vi "动态优化复测判定2.vi"(10 "T1-T2":dbl[](array[numeric]) format="%#.6f", 11 "Vres":dbl[](array[numeric]) format="%#.6f") -> (3 "结果1":bool)   [LabVIEW 2020]
uses:
  Global_Variable/Global.vi
  Global_Variable/A180648.vi
  <userlib>/_MGI/1D Array/MGI Average/MGI Average (DBL[]).vi
panel:
  out "结果2":bool
  out "结果3":bool
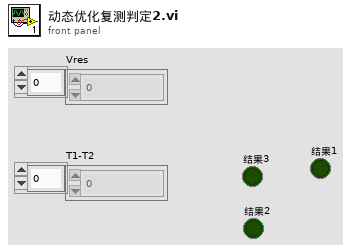
[diagram p1: front panel]
types:
  T1 = cluster{"主副信号合格范围":cluster{"单位":string, "下限":dbl, "上限":dbl}, "可信度合格范围":cluster{"单位":string, "下限":dbl, "上限":dbl}, "主副信号差差值":cluster{"单位":string, "下限":dbl, "上限":dbl}, "静态T1-T2范围":cluster{"单位":string, "下限":dbl, "上限":dbl}, "静态T1-T2偏差范围":cluster{"单位":string, "下限":dbl, "上限":dbl}}
  T2 = cluster{"曲线范围":cluster{"单位":string, "角度下限":dbl, "角度上限":dbl}}
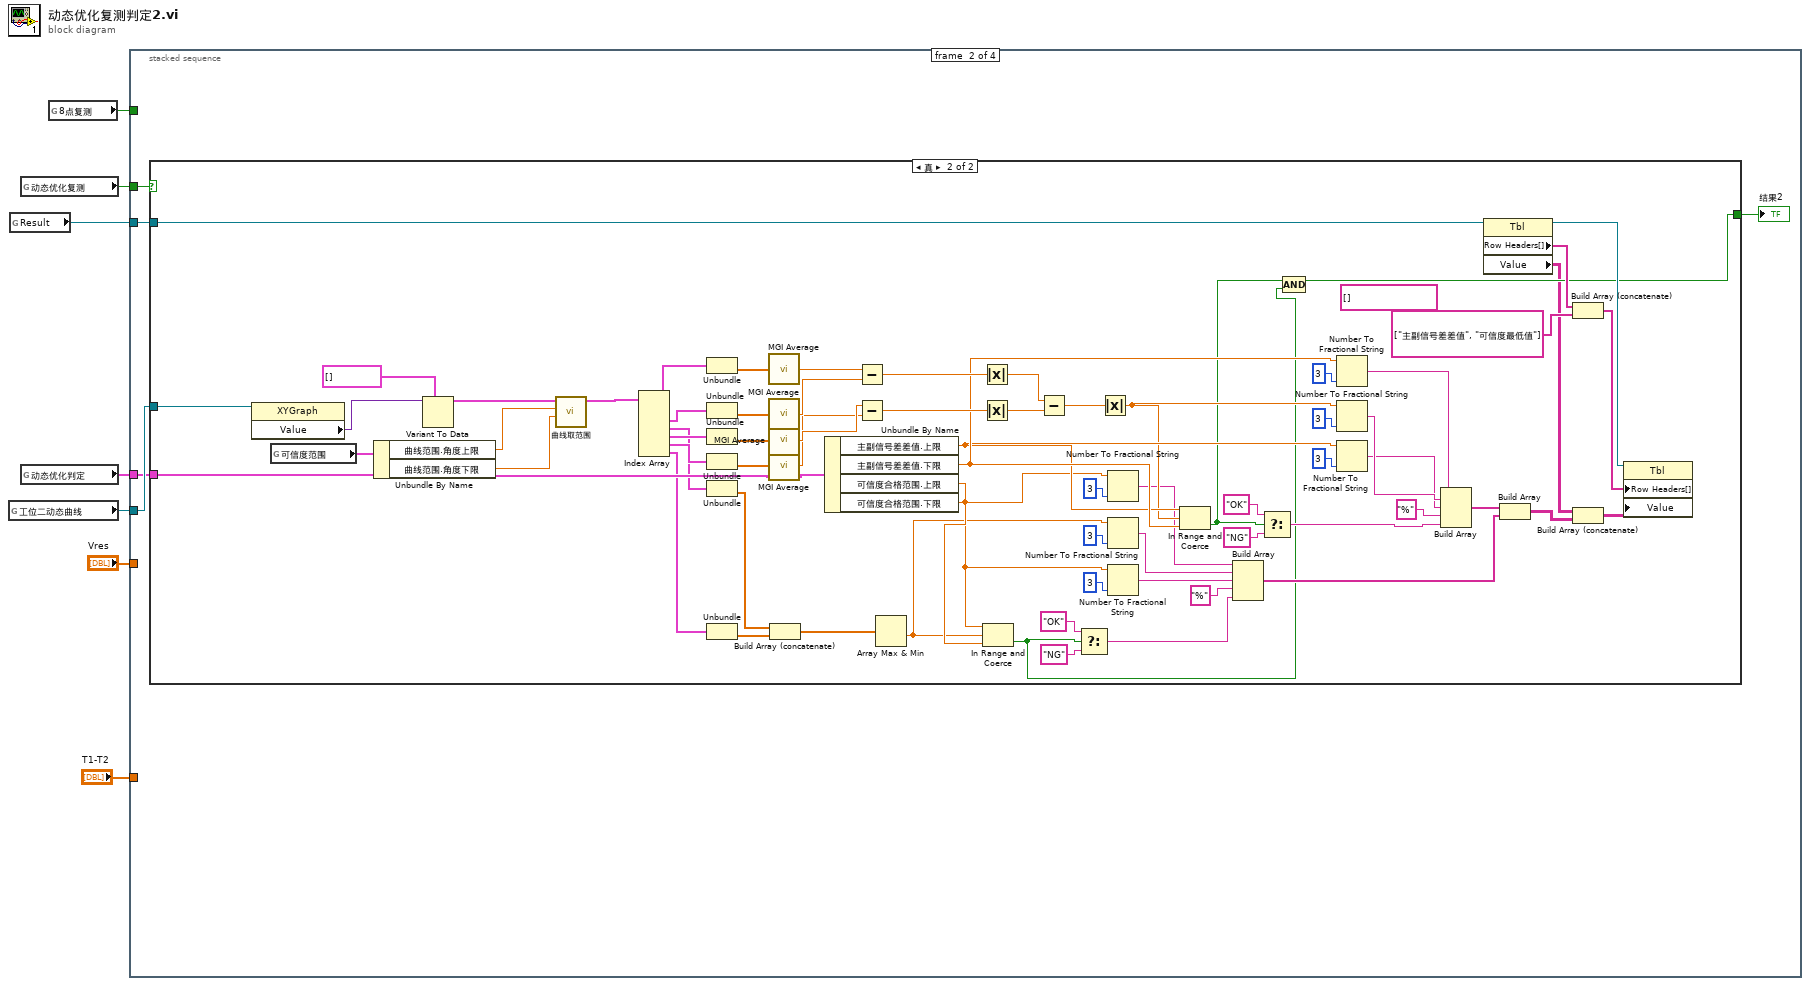
[diagram p0: block diagram]
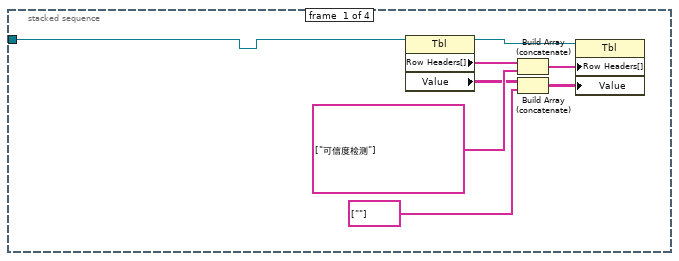
[diagram p2: hidden frame]
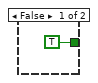
[diagram p3: hidden frame]
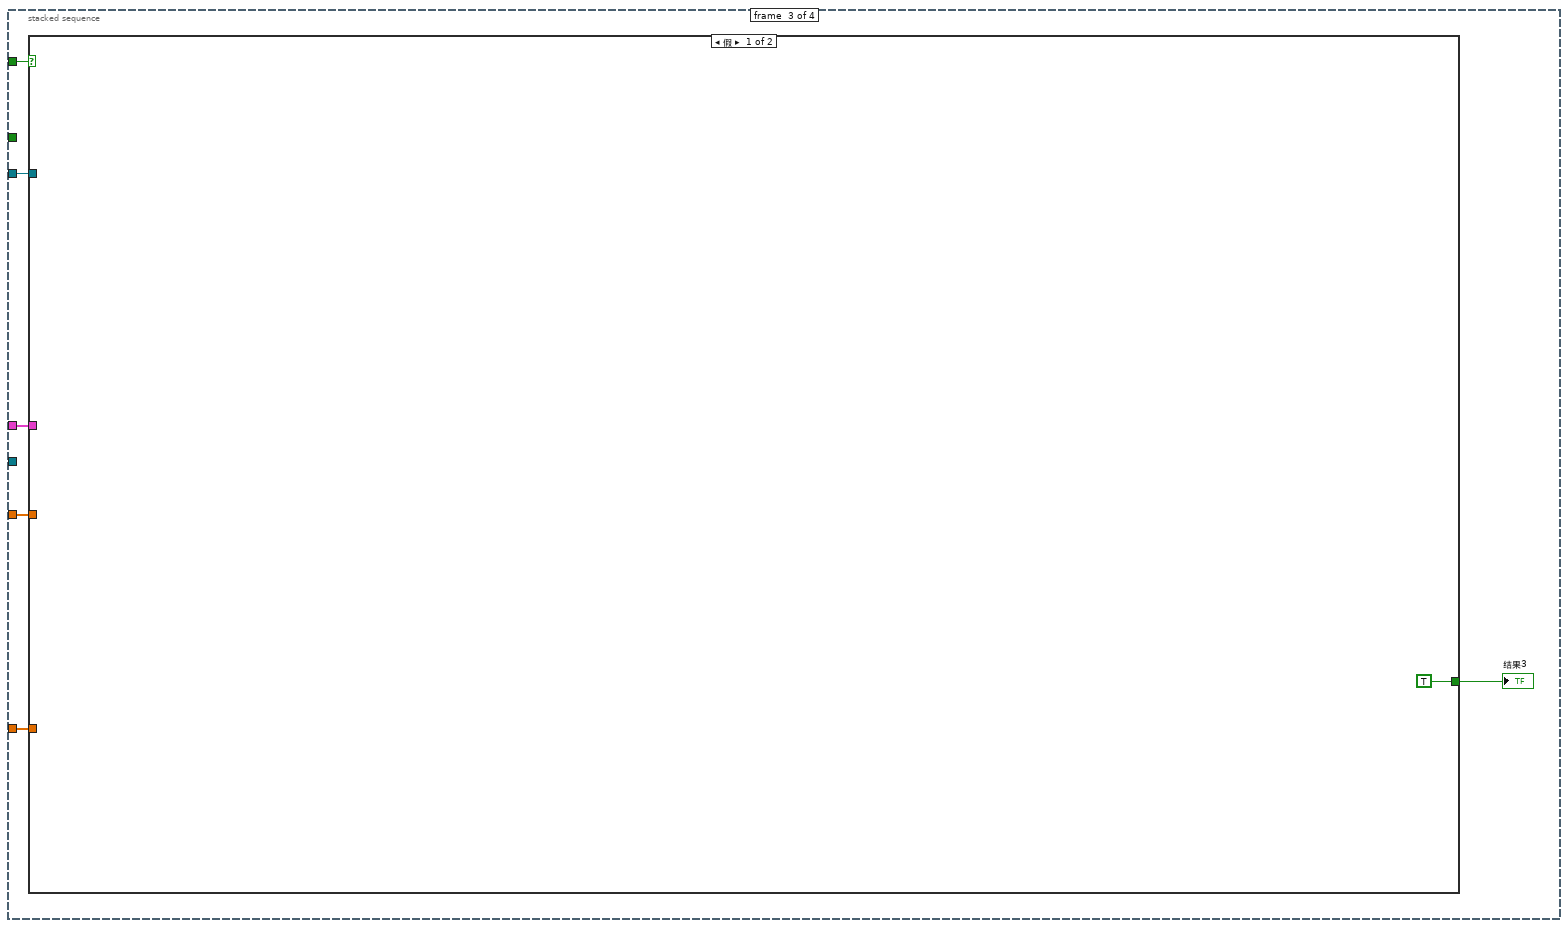
[diagram p4: hidden frame]
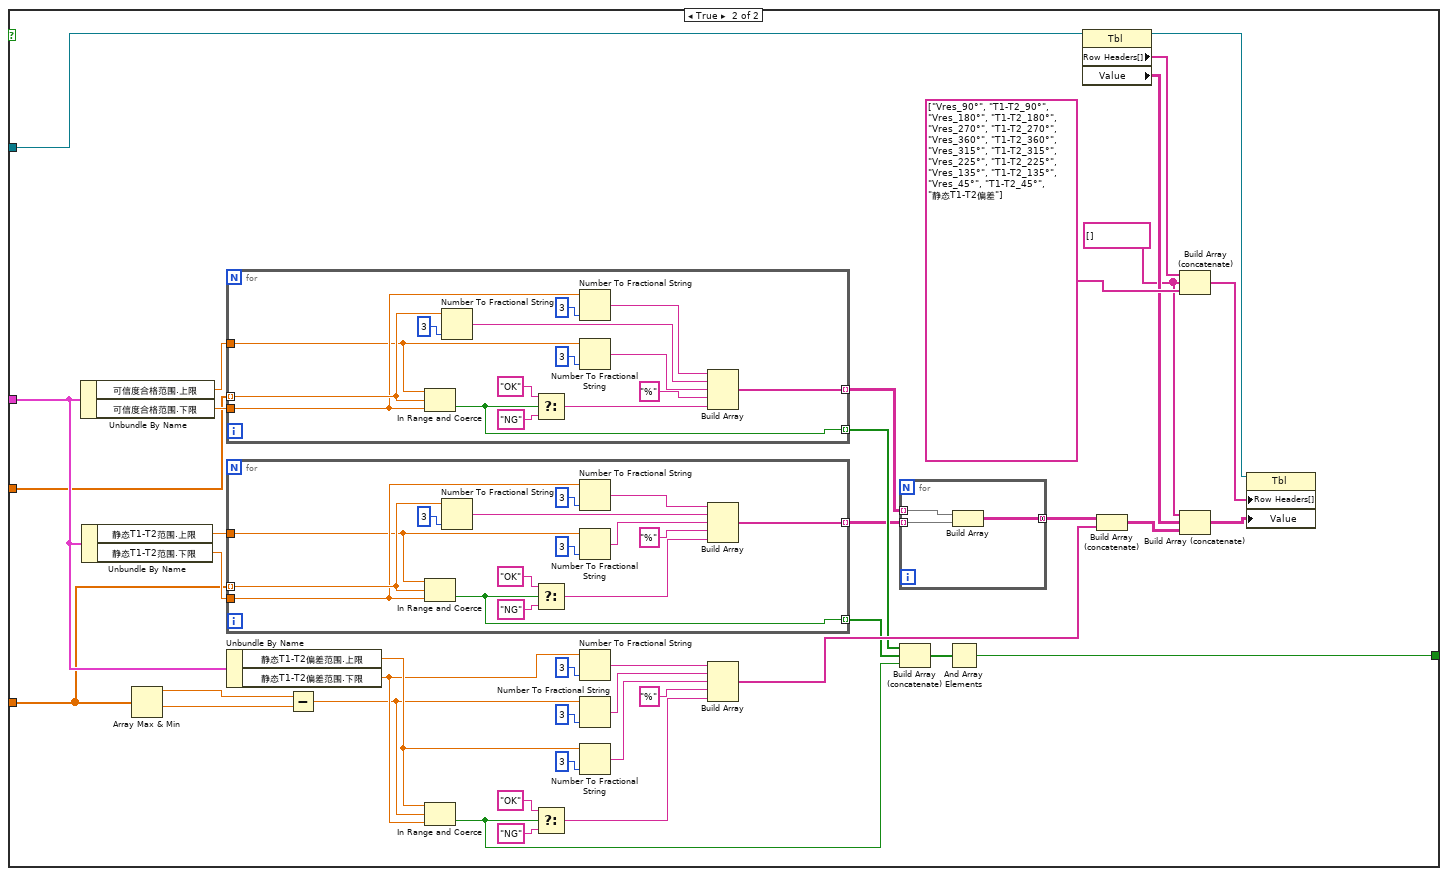
[diagram p5: hidden frame]
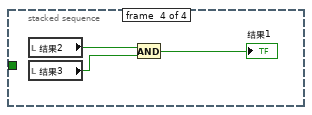
[diagram p6: hidden frame]
diagram:
  n1 = global read "A180648.vi" "工位二动态曲线"() -> (w6:refnum<vi>)
  n2 = global read "Global.vi" "Result"() -> (w1:refnum<vi>)
  n3 = global read "Global.vi" "动态优化复测"() -> (w3:bool)
  n4 = global read "Global.vi" "动态优化判定"() -> (w7:T1)
  n5 = global read "Global.vi" "8点复测"() -> (w2:bool)
  n6 = stacked-sequence {
    tunnel: w1 -> [w8 w20 w97 _]
    tunnel: w7 -> [_ w18 w96 _]
    tunnel: w6 -> [_ w19 _ _]
    tunnel: "Vres" -> [_ _ w95 _]
    tunnel: "T1-T2" -> [_ _ w94 _]
    tunnel: w3 -> [_ w17 _ _]
    tunnel: w2 -> [_ _ w93 _]
    frame #0 {
      n7 = property class="Tbl"(reference=w8) -> (reference out=w15:refnum<vi>, "Row Headers[]"=w14:string[], "Value"=w11:string[][])  [unwired: 1 in, 1 out]
      n8 = Build Array (concatenate)(w14, string[] ["可信度检测"] ("行首字符串[]")) -> (w12:string[])
      n9 = Build Array (concatenate)(w11, string[] [""] ("元素")) -> (w10:string[][])
      n10 = property class="Tbl"(reference=w15, "Row Headers[]"=w12, "Value"=w10) -> ()  [unwired: 1 in, 2 out]
    }
    frame #1 {
      n11 = case shown="真" w17 {
        tunnel: w20 -> [_ w86]
        tunnel: w19 -> [_ w85]
        tunnel: w18 -> [_ w58]
        tunnel: [TRUE w30] -> w16
        frame False {
        }
        frame True {
          (unwired) string[] [] ("行首字符串[]")
          n12 = property class="XYGraph"(reference=w85) -> ("Value"=w84:variant)  [unwired: 1 in, 2 out]
          n13 = global read "Global.vi" "可信度范围"() -> (w24:T2)
          n14 = Unbundle By Name(w24) -> ("曲线范围.角度上限"=w23:dbl, "曲线范围.角度下限"=w22:dbl)
          n15 = Variant To Data(type=cluster{dbl[], dbl[]}[] [], Variant=w84) -> (data=w26:cluster{dbl[], dbl[]}[])  [unwired: 1 in, 1 out]
          n16 = call "曲线取范围.vi"("下限"=w22, "上限"=w23, "曲线In"=w26) -> ("曲线Out"=w25:cluster{"X":dbl[], "Y":dbl[]}[])  [unwired: 8 in]
          n17 = Index Array(array=w25) -> (element #1=w82:cluster{"X":dbl[], "Y":dbl[]}, element #2=w81:cluster{"X":dbl[], "Y":dbl[]}, element #3=w49:cluster{"X":dbl[], "Y":dbl[]}, element #4=w80:cluster{"X":dbl[], "Y":dbl[]}, element #5=w79:cluster{"X":dbl[], "Y":dbl[]}, element #6=w48:cluster{"X":dbl[], "Y":dbl[]})  [unwired: 6 in]
          n18 = Unbundle(w82) -> ("Y"=w75:dbl[])  [unwired: 1 out]
          n19 = Unbundle(w81) -> ("Y"=w76:dbl[])  [unwired: 1 out]
          n20 = Unbundle(w80) -> ("Y"=w78:dbl[])  [unwired: 1 out]
          n21 = Unbundle(w79) -> ("Y"=w77:dbl[])  [unwired: 1 out]
          n22 = Unbundle(w49) -> ("Y"=w46:dbl[])  [unwired: 1 out]
          n23 = Unbundle(w48) -> ("Y"=w47:dbl[])  [unwired: 1 out]
          n24 = call-poly <userlib>:"MGI Average.vi"("Double[]"=w75) -> ("Average"=w56:dbl)  [unwired: 1 in]
          n25 = call-poly <userlib>:"MGI Average.vi"("Double[]"=w76) -> ("Average"=w55:dbl)  [unwired: 1 in]
          n26 = call-poly <userlib>:"MGI Average.vi"("Double[]"=w78) -> ("Average"=w54:dbl)  [unwired: 1 in]
          n27 = call-poly <userlib>:"MGI Average.vi"("Double[]"=w77) -> ("Average"=w53:dbl)  [unwired: 1 in]
          n28 = Build Array (concatenate)(w46, w47) -> (w45:dbl[])
          n29 = Unbundle By Name(w58) -> ("主副信号差差值.上限"=w67:dbl, "主副信号差差值.下限"=w70:dbl, "可信度合格范围.上限"=w37:dbl, "可信度合格范围.下限"=w39:dbl)
          n30 = Subtract(x=w56, y=w55) -> (x-y=w74:dbl)
          n31 = Subtract(x=w54, y=w53) -> (x-y=w73:dbl)
          n32 = Array Max & Min(array=w45) -> (min value=w38:dbl)  [unwired: 3 out]
          n33 = Absolute Value(x=w74) -> (abs(x)=w52:dbl)
          n34 = Absolute Value(x=w73) -> (abs(x)=w51:dbl)
          n35 = In Range and Coerce(upper limit=w37, x=w38, lower limit=w39) -> (In Range?=w29:bool)  [unwired: 1 out]
          n36 = Subtract(x=w52, y=w51) -> (x-y=w72:dbl)
          n37 = Select(t="OK", s=w29, f="NG") -> (s? t:f=w32:string)
          n38 = Absolute Value(x=w72) -> (abs(x)=w57:dbl)
          n39 = Number To Fractional String(number=w39, precision (6)=i16 3 ("精度(6)")) -> (F-format string=w36:string)  [unwired: 2 in]
          n40 = Number To Fractional String(number=w38, precision (6)=i16 3 ("精度(6)")) -> (F-format string=w35:string)  [unwired: 2 in]
          n41 = Number To Fractional String(number=w37, precision (6)=i16 3 ("精度(6)")) -> (F-format string=w34:string)  [unwired: 2 in]
          n42 = In Range and Coerce(upper limit=w67, x=w57, lower limit=w70) -> (In Range?=w50:bool)  [unwired: 1 out]
          n43 = Build Array(w36, w35, w34, "%" ("元素"), w32) -> (w31:string[])
          n44 = Select(t="OK", s=w50, f="NG") -> (s? t:f=w60:string)
          n45 = Compound Arithmetic op=AND ("复合运算")(w50, w29) -> (w30:bool)
          n46 = Number To Fractional String(number=w70, precision (6)=i16 3 ("精度(6)")) -> (F-format string=w66:string)  [unwired: 2 in]
          n47 = Number To Fractional String(number=w57, precision (6)=i16 3 ("精度(6)")) -> (F-format string=w65:string)  [unwired: 2 in]
          n48 = Number To Fractional String(number=w67, precision (6)=i16 3 ("精度(6)")) -> (F-format string=w64:string)  [unwired: 2 in]
          n49 = Build Array(w66, w65, w64, "%" ("元素"), w60) -> (w59:string[])
          n50 = property class="Tbl"(reference=w86) -> (reference out=w91:refnum<vi>, "Row Headers[]"=w90:string[], "Value"=w27:string[][])  [unwired: 1 in, 1 out]
          n51 = Build Array(w59, w31) -> (w87:string[][])
          n52 = Build Array (concatenate)(w90, string[] ["主副信号差差值", "可信度最低值"] ("行首字符串[]")) -> (w89:string[])
          n53 = Build Array (concatenate)(w27, w87) -> (w88:string[][])
          n54 = property class="Tbl"(reference=w91, "Row Headers[]"=w89, "Value"=w88) -> ()  [unwired: 1 in, 2 out]
        }
      }
      "结果2" <- w16
    }
    frame #2 {
      n55 = case shown="假" w93 {
        tunnel: w97 -> [_ w131]
        tunnel: w96 -> [_ w114]
        tunnel: w95 -> [_ w103]
        tunnel: w94 -> [_ w102]
        tunnel: [TRUE w101] -> w92
        frame False {
        }
        frame True {
          w99 = string[] [] ("数组")
          n56 = Unbundle By Name(w114) -> ("可信度合格范围.上限"=w121:dbl, "可信度合格范围.下限"=w120:dbl)
          n57 = Unbundle By Name(w114) -> ("静态T1-T2范围.上限"=w112:dbl, "静态T1-T2范围.下限"=w113:dbl)
          n58 = Array Max & Min(array=w102) -> (max value=w111:dbl, min value=w110:dbl)  [unwired: 2 out]
          n59 = for {
            tunnel: w103 -> [w170] mode=indexing
            tunnel: w121 -> [w166]
            tunnel: w120 -> [w167]
            tunnel: [w158] -> w106 mode=indexing
            tunnel: [w157] -> w108 mode=indexing
            n60 = In Range and Coerce(upper limit=w166, x=w170, lower limit=w167) -> (In Range?=w157:bool)  [unwired: 1 out]
            n61 = Number To Fractional String(number=w170, precision (6)=i16 3 ("精度(6)")) -> (F-format string=w164:string)  [unwired: 2 in]
            n62 = Select(t="OK", s=w157, f="NG") -> (s? t:f=w159:string)
            n63 = Number To Fractional String(number=w167, precision (6)=i16 3 ("精度(6)")) -> (F-format string=w165:string)  [unwired: 2 in]
            n64 = Number To Fractional String(number=w166, precision (6)=i16 3 ("精度(6)")) -> (F-format string=w163:string)  [unwired: 2 in]
            n65 = Build Array(w165, w164, w163, "%", w159) -> (w158:string[])
          }
          n66 = for {
            tunnel: w102 -> [w155] mode=indexing
            tunnel: w112 -> [w151]
            tunnel: w113 -> [w152]
            tunnel: [w143] -> w105 mode=indexing
            tunnel: [w142] -> w107 mode=indexing
            n67 = In Range and Coerce(upper limit=w151, x=w155, lower limit=w152) -> (In Range?=w142:bool)  [unwired: 1 out]
            n68 = Number To Fractional String(number=w155, precision (6)=i16 3 ("精度(6)")) -> (F-format string=w149:string)  [unwired: 2 in]
            n69 = Select(t="OK", s=w142, f="NG") -> (s? t:f=w144:string)
            n70 = Number To Fractional String(number=w152, precision (6)=i16 3 ("精度(6)")) -> (F-format string=w150:string)  [unwired: 2 in]
            n71 = Number To Fractional String(number=w151, precision (6)=i16 3 ("精度(6)")) -> (F-format string=w148:string)  [unwired: 2 in]
            n72 = Build Array(w150, w149, w148, "%", w144) -> (w143:string[])
          }
          n73 = Unbundle By Name(w114) -> ("静态T1-T2偏差范围.上限"=w119:dbl, "静态T1-T2偏差范围.下限"=w117:dbl)
          n74 = Subtract(x=w111, y=w110) -> (x-y=w109:dbl)
          n75 = In Range and Coerce(upper limit=w119, x=w109, lower limit=w117) -> (In Range?=w123:bool)  [unwired: 1 out]
          n76 = Select(t="OK", s=w123, f="NG") -> (s? t:f=w128:string)
          n77 = Number To Fractional String(number=w117, precision (6)=i16 3 ("宽度(-)")) -> (F-format string=w116:string)  [unwired: 2 in]
          n78 = Number To Fractional String(number=w109, precision (6)=i16 3 ("宽度(-)")) -> (F-format string=w125:string)  [unwired: 2 in]
          n79 = Number To Fractional String(number=w119, precision (6)=i16 3 ("精度(6)")) -> (F-format string=w124:string)  [unwired: 2 in]
          n80 = Build Array(w116, w125, w124, "%" ("元素"), w128) -> (w115:string[])
          n81 = for {
            tunnel: w106 -> [w141] mode=indexing
            tunnel: w105 -> [w140] mode=indexing
            tunnel: [w139] -> w104 mode=concatenating
            n82 = Build Array(w141, w140) -> (w139:string[][])
          }
          n83 = Build Array (concatenate)(w108, w107, w123) -> (w138:bool[])
          n84 = And Array Elements(Boolean array=w138) -> (logical AND=w101:bool)
          n85 = property class="Tbl"(reference=w131) -> (reference out=w137:refnum<vi>, "Row Headers[]"=w136:string[], "Value"=w100:string[][])  [unwired: 1 in, 1 out]
          n86 = Build Array (concatenate)(w104, w115) -> (w132:string[][])
          n87 = Build Array (concatenate)(w136, w99, string[] ["Vres_90°", "T1-T2_90°", "Vres_180°", "T1-T2_180°", "Vres_270°", "T1-T2_270°", "Vres_360°", "T1-T2_360°", "Vres_315°", "T1-T2_315°", "Vres_225°", "T1-T2_225°", "Vres_135°", "T1-T2_135°", "Vres_45°", "T1-T2_45°", "静态T1-T2偏差"] ("行首字符串[]")) -> (w134:string[])
          n88 = Build Array (concatenate)(w99, w100, w132) -> (w133:string[][])
          n89 = property class="Tbl"(reference=w137, "Row Headers[]"=w134, "Value"=w133) -> ()  [unwired: 1 in, 2 out]
        }
      }
      "结果3" <- w92
    }
    frame #3 {
      n90 = local read "结果2"() -> (w174:bool)
      n91 = local read "结果3"() -> (w173:bool)
      n92 = And(x=w174, y=w173) -> (x .and. y?=→"结果1":bool)
    }
  }
